vi "Obj_Position.vi"(4 "error in":errorcluster, 7 "Ctl Refnum":refnum<vi>) -> (0 "error out":errorcluster, 2 "Position":T1)   [LabVIEW 8.6]
panel:
  in  "Button":bool
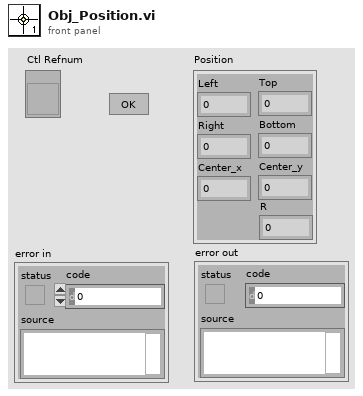
[diagram p1: front panel]
types:
  T1 = cluster{"Left":i32, "Right":i32, "Top":i32, "Bottom":i32, "Center_x":i32, "Center_y":i32, "R":i32}
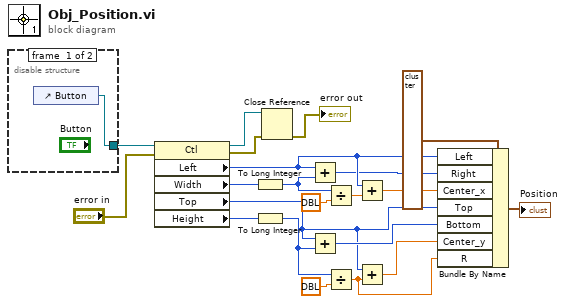
[diagram p0: block diagram]
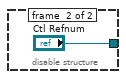
[diagram p2: hidden frame]
diagram:
  n1 = disable-structure shown="Enabled" {
    disable-tunnel: [w22 "Ctl Refnum"] -> w20
    frame #0 {
      n2 = control-ref of="Button"() -> (w22:refnum<vi>)
    }
    frame #1 {
    }
  }
  n3 = property class="Ctl"(reference=w20, error in="error in") -> (reference out=w1:refnum<vi>, error out=w3:errorcluster, "Left"=w11:i32, "Width"=w7:u32, "Top"=w12:i32, "Height"=w10:u32)
  n4 = To Long Integer(number=w7) -> (32bit integer=w8:i32)
  n5 = To Long Integer(number=w10) -> (32bit integer=w9:i32)
  n6 = Close Reference(reference=w1, error in (no error)=w3) -> (error out=→"error out":errorcluster)
  n7 = Add(x=w11, y=w8) -> (x+y=w6:i32)
  n8 = Add(x=w12, y=w9) -> (x+y=w13:i32)
  n9 = Divide(x=w8, y=dbl ?) -> (x/y=w18:dbl)
  n10 = Divide(x=w9, y=dbl ?) -> (x/y=w4:dbl)
  n11 = Add(x=w11, y=w18) -> (x+y=w5:dbl)
  n12 = Add(x=w12, y=w4) -> (x+y=w14:dbl)
  n13 = Bundle By Name(cluster=T1 ? ("Position"), "Left"=w11, "Right"=w6, "Center_x"=w5, "Top"=w12, "Bottom"=w13, "Center_y"=w14, "R"=w4) -> (→"Position":T1)
